vi "q1 sum odd numbers for loop.vi"() -> ()   [LabVIEW 2025]
panel:
  out "sum of n\nodd numbers\n(if)":dbl
  in  "n":dbl
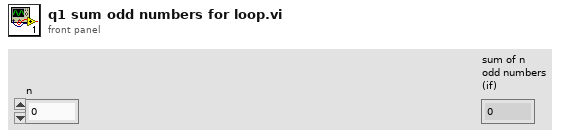
[diagram p1: front panel]
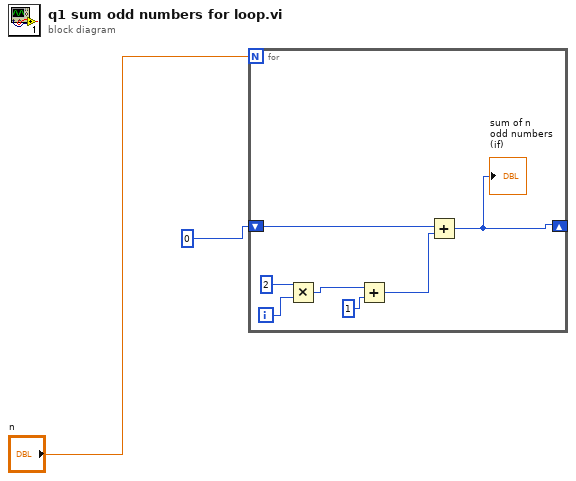
[diagram p0: block diagram]
diagram:
  n1 = for {
    N: "n" -> [_]
    shift-right: [w3] -> _
    shift-left: 0 -> [w7]
    i -> [w8]
    n2 = Multiply(x=2, y=w8) -> (x*y=w6:i32)
    n3 = Add(x=w6, y=1) -> (x+y=w4:i32)
    n4 = Add(x=w7, y=w4) -> (x+y=w3:i32)
    "sum of n\nodd numbers\n(if)" <- w3
  }
